vi "_TangoAttributeEventGroupKill.vi"(1 "error in":errorcluster, 2 "attribute event ref.":T1) -> (0 "error out":errorcluster)   [LabVIEW 2014, in "tango.lvlib"]
uses:
  tango.lvlib
  Common VIs/Typedefs/_AttributeEventRef.ctl
  Common VIs/Typedefs/_AttributeValue_t.ctl
  Common VIs/Typedefs/_AttributeQuality_t.ctl
  Common VIs/Typedefs/_AttributeDataType_t.ctl
  tango_binding.so
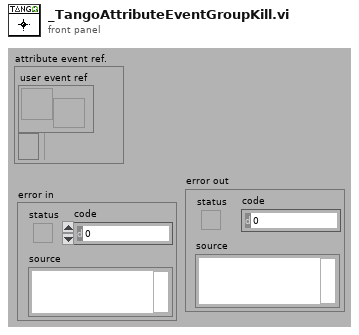
[diagram p1: front panel]
types:
  T1 = typedef "tango.lvlib/_AttributeEventRef.ctl" = cluster{"user event ref":refnum<user-event>, "user event reg refnum":refnum<event-registration>}
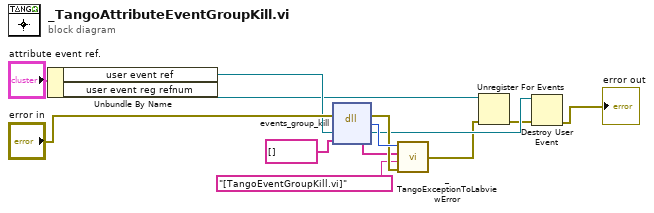
[diagram p0: block diagram]
diagram:
  n1 = Unbundle By Name("attribute event ref.") -> ("user event ref"=w6:refnum<user-event>, "user event reg refnum"=w4:refnum<event-registration>)
  n2 = dll-call lib="tango_binding.*" fn="events_group_kill"(error in="error in", "event refnum"=w6, "error_stack"=string[] []) -> (error out=w11:errorcluster, "return type"=w12:i32, "event refnum"=w5:refnum<user-event>, "error_stack"=w10:string[])  [unwired: 2 in, 1 out]
  n3 = call "_TangoExceptionToLabviewError.vi"("error in"=w11, "location"="[TangoEventGroupKill.vi]", "error stack"=w10, "error code"=w12) -> ("error out"=w3:errorcluster)
  n4 = Unregister For Events(event registration refnum=w4, error in=w3) -> (error out=w2:errorcluster)
  n5 = Destroy User Event(user event=w5, error in=w2) -> (error out=→"error out":errorcluster)
